vi "VectorField1010.vi"   [LabVIEW 2013]
uses:
  <vilib>/Heliosphere Research LLC/Advanced Plotting Toolkit/api_plotting/VectorFieldProperties.ctl
  <vilib>/Heliosphere Research LLC/Advanced Plotting Toolkit/typedefs/PlotColor.ctl
  <vilib>/Heliosphere Research LLC/Advanced Plotting Toolkit/properties/Colormap.ctl
  <vilib>/Heliosphere Research LLC/Advanced Plotting Toolkit/properties/Colormap_Map.ctl
  <vilib>/Heliosphere Research LLC/Advanced Plotting Toolkit/properties/Colormap_Scaling.ctl
  <vilib>/Heliosphere Research LLC/Advanced Plotting Toolkit/properties/Display.ctl
  <vilib>/Heliosphere Research LLC/Advanced Plotting Toolkit/Advanced Plotting Toolkit.lvlib
types:
  T1 = typedef "Advanced Plotting Toolkit.lvlib/PlotColor.ctl" = u32
  T2 = typedef "Advanced Plotting Toolkit.lvlib/VectorFieldProperties.ctl" = cluster{"Color":T1, "Arrow Scale":dbl, "Colormap":T3, "Display":T6}
  T3 = typedef "Advanced Plotting Toolkit.lvlib/Colormap.ctl" = cluster{"Map":T4, "Value Min":dbl, "Value Max":dbl, "Scaling":T5, "Reverse":bool}
  T4 = typedef "Advanced Plotting Toolkit.lvlib/Colormap_Map.ctl" = enum16{"Automatic", "Rainbow", "Hot and Cold", "White-Black", "White-Blue", "White-Green", "White-Red", "Fire", "Water", "Earth", "Air", "Pastel", "Banded", "Stepped"}
  T5 = typedef "Advanced Plotting Toolkit.lvlib/Colormap_Scaling.ctl" = enum16{"Default"}
  T6 = typedef "Advanced Plotting Toolkit.lvlib/Display.ctl" = cluster{"Alpha":dbl, "Z Order":dbl}
  T7 = typedef "Advanced Plotting Toolkit.lvlib/PlotID.ctl" = i32
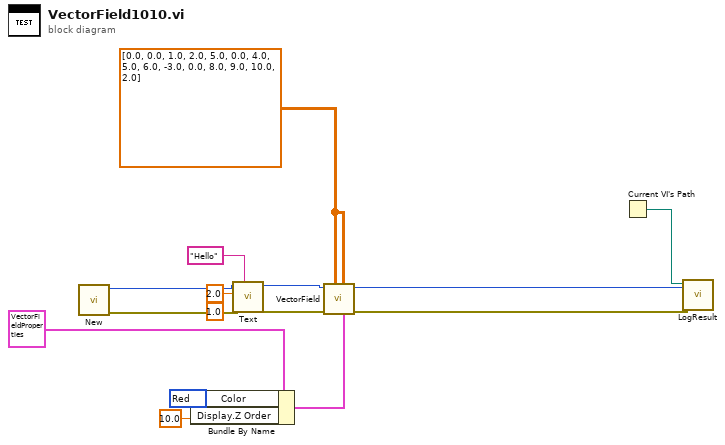
[diagram p0: block diagram]
diagram:
  w2 = T1 16711680 items=["Automatic"=2147483647, "Black"=0, "White"=16777215, "Red"=16711680, "Green"=2263842, "Blue"=255, "Cyan"=65535, "Magenta"=16711935, "Yellow"=16776960] ("Color")
  w14 = dbl[][] [[0.0, 0.0, 1.0, 2.0, 5.0], [0.0, 4.0, 5.0, 6.0, -3.0], [0.0, 8.0, 9.0, 10.0, 2.0]] ("Data")
  n1 = call <vilib>:"New.vi"() -> ("error out"=w7:errorcluster, "Plot ID"=w9:T7)  [unwired: 10 in]
  n2 = Bundle By Name(cluster=T2 {"Color"=2147483647, "Arrow Scale"=nan, "Colormap"={"Map"=enum."Automatic", "Value Min"=nan, "Value Max"=nan, "Scaling"=enum."Default", "Reverse"=FALSE}, "Display"={"Alpha"=nan, "Z Order"=nan}} ("Vector Field Properties"), "Color"=w2, "Display.Z Order"=10.0) -> (w10:T2)
  n3 = call <vilib>:"Text.vi"("Text"="Hello", "error in (no error)"=w7, "Y Position"=1.0, "X Position"=2.0, "Plot ID"=w9) -> ("error out"=w6:errorcluster, "Plot ID Out"=w8:T7)  [unwired: 5 in]
  n4 = call <vilib>:"VectorField.vi"("Properties"=w10, "Y Vector Component"=w14, "X Vector Component"=w14, "error in (no error)"=w6, "Plot ID"=w8) -> ("error out"=w12:errorcluster, "Plot ID Out"=w13:T7)  [unwired: 5 in]
  n5 = Current VI's Path() -> (path=w15:path)
  n6 = call "LogResult.vi"("Test Result"=w12, "Test Artifact"=w13, "VI Path"=w15) -> ()  [unwired: 9 in]
